vi "Compare VI Folders.vi"(8 "error in (no error)":errorcluster, 9 "VI Comparison Options":T1={"VI Attributes?"=TRUE, "Front Panel"=FALSE, "Front Panel Position/Size"=FALSE, "Block Diagram"=TRUE, "Block Diagram Cosmetic"=FALSE, "Block Diagram Position/Size"=FALSE}, 10 "Folder 2":path, 11 "Folder 1":path) -> (0 "error out":errorcluster, 3 "VIs Modiifed[]":path[](array[path]))   [LabVIEW 2014, in "SLL Utilities.lvlib"]
uses:
  SLL Utilities.lvlib
  _Typedefs/VI Comparison Options.ctl
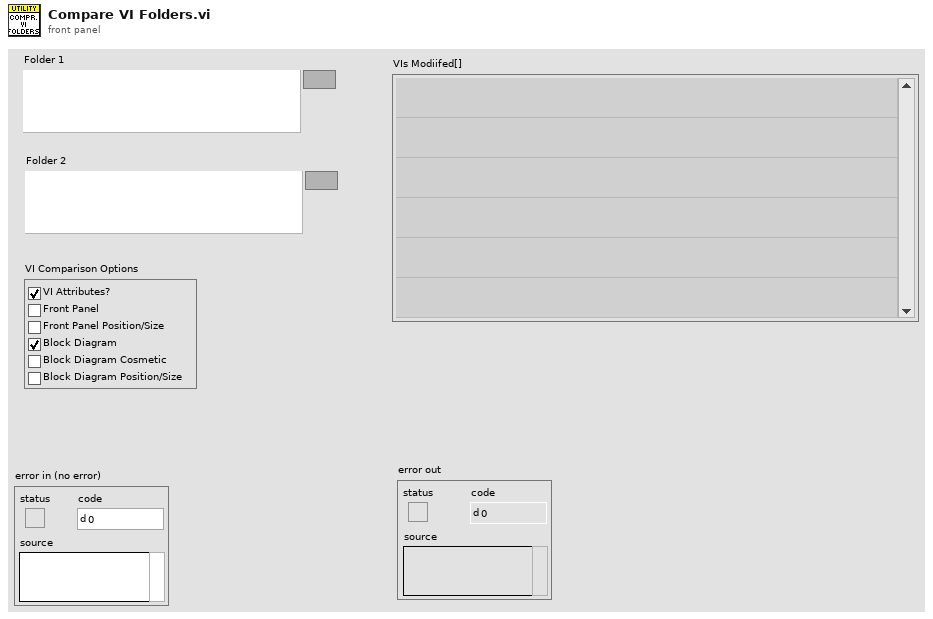
[diagram p1: front panel]
types:
  T1 = typedef "SLL Utilities.lvlib/VI Comparison Options.ctl" = cluster{"VI Attributes?":bool, "Front Panel":bool, "Front Panel Position/Size":bool, "Block Diagram":bool, "Block Diagram Cosmetic":bool, "Block Diagram Position/Size":bool}
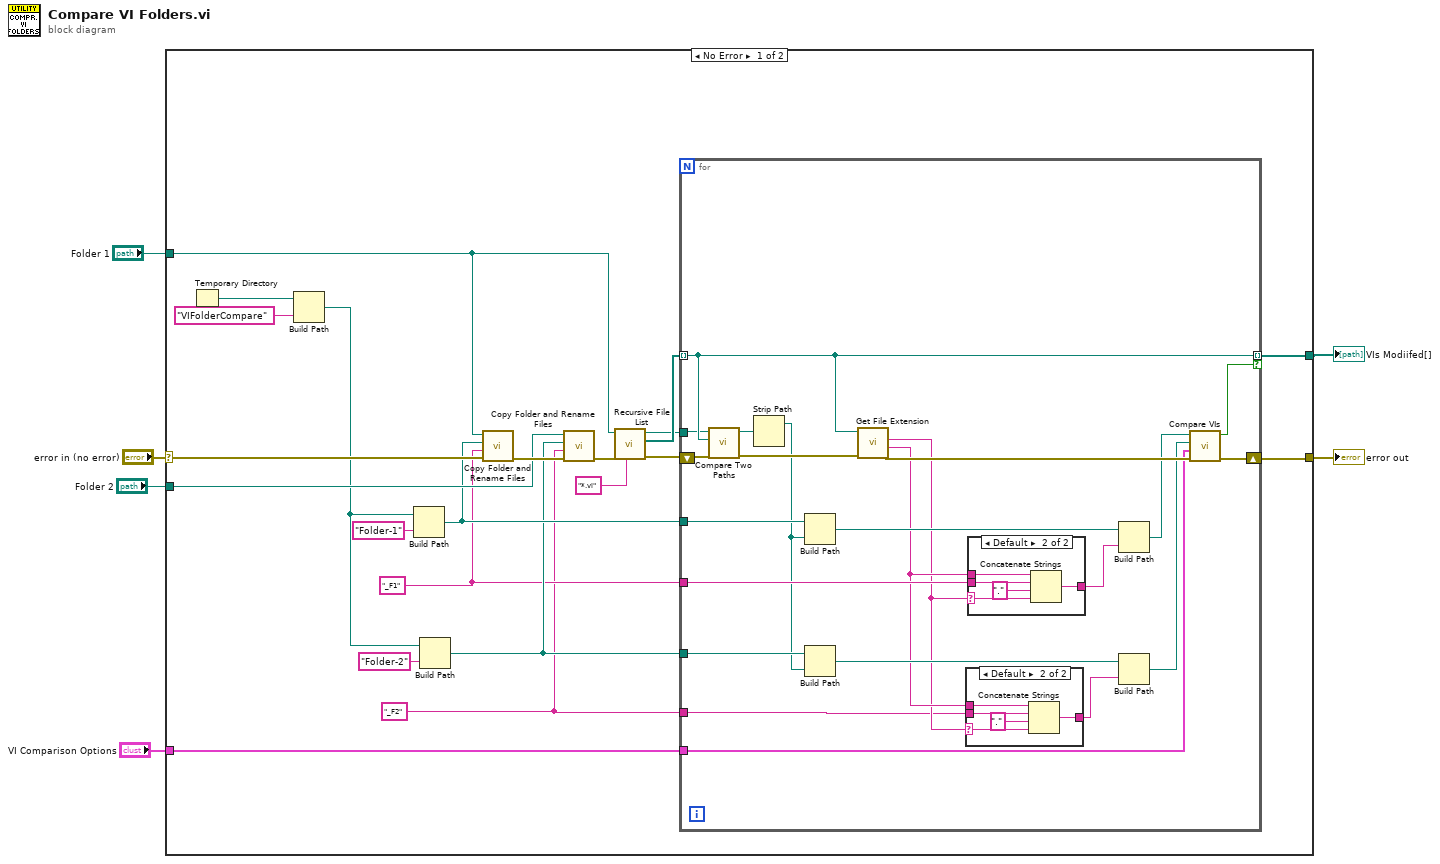
[diagram p0: block diagram]
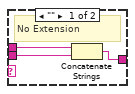
[diagram p2: hidden frame]
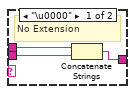
[diagram p3: hidden frame]
diagram:
  n1 = case shown="No Error" "error in (no error)" {
    selector: "error in (no error)" -> [w27 w66]
    tunnel: [w11 w66] -> w5
    tunnel: "Folder 1" -> [w16 _]
    tunnel: "Folder 2" -> [w22 _]
    tunnel: [w9 _] -> w2
    tunnel: "VI Comparison Options" -> [w8 _]
    frame No Error {
      w12 = "_F2" ("File Name Suffix")
      w13 = "_F1" ("File Name Suffix")
      n2 = Temporary Directory() -> (w26:path)
      n3 = Build Path(base path=w26, name or relative path="VIFolderCompare") -> (appended path=w20:path)
      n4 = Build Path(base path=w20, name or relative path="Folder-1") -> (appended path=w15:path)
      n5 = Build Path(base path=w20, name or relative path="Folder-2") -> (appended path=w14:path)
      n6 = call "Copy Folder and Rename Files.vi"("error in (no error)"=w27, "File Name Suffix"=w13, "Destination Folder"=w15, "Source Folder"=w16) -> ("error out"=w23:errorcluster)  [unwired: 7 in]
      n7 = call "Copy Folder and Rename Files.vi"("error in (no error)"=w23, "File Name Suffix"=w12, "Destination Folder"=w14, "Source Folder"=w22) -> ("error out"=w19:errorcluster)  [unwired: 7 in]
      n8 = call <vilib>:"Recursive File List.vi"("pattern"="*.vi", "error in (no error)"=w19, "Folder Path"=w16) -> ("error out"=w18:errorcluster, "All Files in Dir"=w17:path[], "dup Folder Path"=w10:path)  [unwired: 4 in, 2 out]
      n9 = for {
        tunnel: w17 -> [w35] mode=indexing
        tunnel: w10 -> [w34]
        tunnel: w15 -> [w48]
        tunnel: w14 -> [w47]
        tunnel: w13 -> [w44]
        tunnel: w12 -> [w29]
        shift-right: [w38] -> w11
        shift-left: w18 -> [w49]
        tunnel: [w35] -> w9 mode=indexing if=w37
        tunnel: w8 -> [w36]
        n10 = call <vilib>:"Compare Two Paths.vi"("error in (no error)"=w49, "Path 2"=w35, "Path 1"=w34) -> ("error out"=w45:errorcluster, "Relative Path from 1 to 2"=w33:path)  [unwired: 5 in, 2 out]
        n11 = Strip Path(path=w33) -> (stripped path=w32:path)  [unwired: 1 out]
        n12 = Build Path(base path=w48, name or relative path=w32) -> (appended path=w43:path)
        n13 = Build Path(base path=w47, name or relative path=w32) -> (appended path=w42:path)
        n14 = call <vilib>:"Get File Extension.vi"("error in (no error)"=w45, "file"=w35) -> ("error out"=w41:errorcluster, "filename without extension"=w31:string, "lowercase file extension"=w30:string)  [unwired: 6 in, 1 out]
        n15 = case shown="Default" w30 {
          selector: w30 -> [_ w53]
          tunnel: [w52 w56] -> w28
          tunnel: w29 -> [w51 w55]
          tunnel: w31 -> [w50 w54]
          frame "" {
            # "No Extension"
            n16 = Concatenate Strings(w50, w51) -> (w52:string)
          }
          frame Default {
            n17 = Concatenate Strings(w54, w55, "." ("string"), w53) -> (w56:string)
          }
        }
        n18 = case shown="Default" w30 {
          selector: w30 -> [_ w61]
          tunnel: [w60 w64] -> w46
          tunnel: w44 -> [w59 w63]
          tunnel: w31 -> [w58 w62]
          frame "\u0000" {
            # "No Extension"
            n19 = Concatenate Strings(w58, w59) -> (w60:string)
          }
          frame Default {
            n20 = Concatenate Strings(w62, w63, "." ("string"), w61) -> (w64:string)
          }
        }
        n21 = Build Path(base path=w43, name or relative path=w46) -> (appended path=w40:path)
        n22 = Build Path(base path=w42, name or relative path=w28) -> (appended path=w39:path)
        n23 = call "Compare VIs.vi"("error in (no error)"=w41, "VI Comparison Options"=w36, "VI Path 2"=w39, "VI Path 1"=w40) -> ("error out"=w38:errorcluster, "Different?"=w37:bool)  [unwired: 6 in]
      }
    }
    frame Error {
    }
  }
  "error out" <- w5
  "VIs Modiifed[]" <- w2
